vi "keepLogBoundsPositive.vi"(10 "Mapping":enum16{"Lin", "Log"}(ring), 11 "AxisBounds in":T1) -> (3 "AxisBounds out":T1)   [LabVIEW 2013]
uses:
  minAndMax.ctl
  AutoManualNumber.ctl
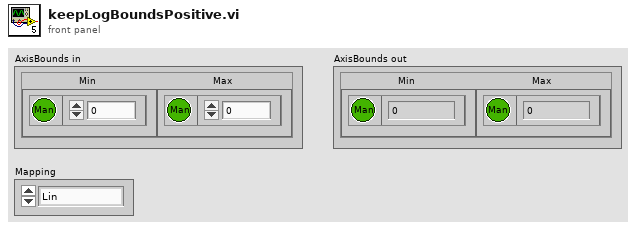
[diagram p1: front panel]
types:
  T1 = typedef "minAndMax.ctl" = cluster{"Min":T2, "Max":T2}
  T2 = typedef "AutoManualNumber.ctl" = cluster{"Auto":bool, "Value":dbl}
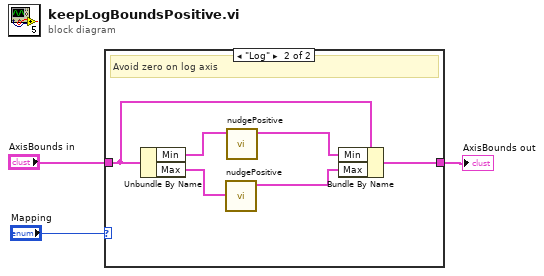
[diagram p0: block diagram]
diagram:
  n1 = case shown="\"Log\"" "Mapping" {
    tunnel: [w4 w5] -> w1
    tunnel: "AxisBounds in" -> [w4 w9]
    frame "Lin", Default {
    }
    frame "Log" {
      # "Avoid zero on log axis"
      n2 = Unbundle By Name(w9) -> ("Min"=w10:T2, "Max"=w7:T2)
      n3 = call "nudgePositive.vi"("Min in"=w7) -> ("Min out"=w6:T2)  [unwired: 10 in]
      n4 = call "nudgePositive.vi"("Min in"=w10) -> ("Min out"=w8:T2)  [unwired: 10 in]
      n5 = Bundle By Name(cluster=w9, "Min"=w8, "Max"=w6) -> (w5:T1)
    }
  }
  "AxisBounds out" <- w1
